vi "Data Ref FGV.vi"(5 "FIFO Idx Qs":T1, 7 "Command":T2=enum."Get", 8 "error in (no error)":errorcluster, 10 "HWOutput Length":i32, 11 "HWInput Length":i32) -> (0 "error out":errorcluster, 2 "HWOutput FIFO Index / Length":i32, 3 "HWInput FIFO Index / Length":i32)   [LabVIEW 2011, in "AIT 1553 Custom Device.lvlib"]
uses:
  AIT 1553 Custom Device.lvlib
  RT Controls/Data Ref FGV Command.ctl
  RT Controls/FIFO Idx Qs.ctl
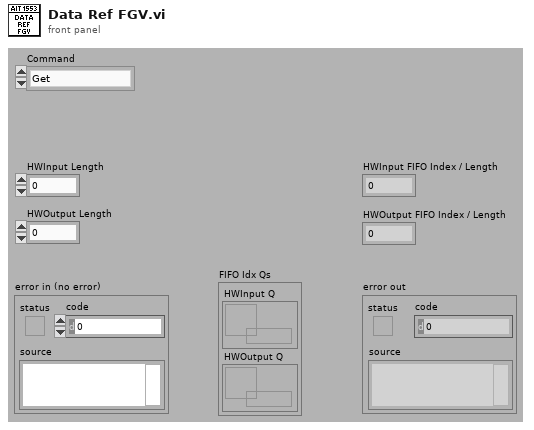
[diagram p1: front panel]
types:
  T1 = typedef "AIT 1553 Custom Device.lvlib/FIFO Idx Qs.ctl" = cluster{"HWInput Q":refnum<queue>, "HWOutput Q":refnum<queue>}
  T2 = typedef "AIT 1553 Custom Device.lvlib/Data Ref FGV Command.ctl" = enum16{"Intialize", "Get", "Update"}
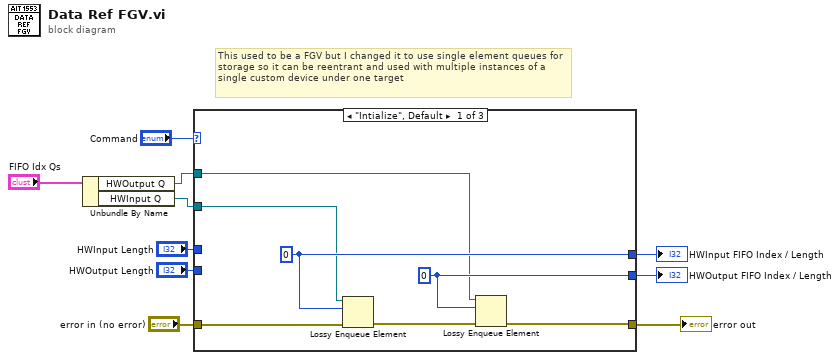
[diagram p0: block diagram]
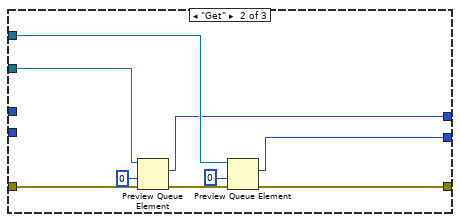
[diagram p2: hidden frame]
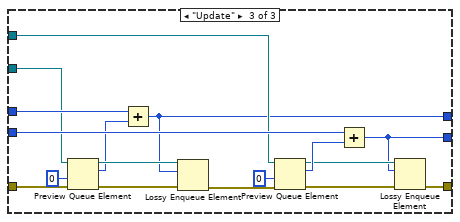
[diagram p3: hidden frame]
diagram:
  # "This used to be a FGV but I changed it to use single element queues for storage so it can be reentrant and used with multiple instances of a single custom device under one target"
  n1 = Unbundle By Name("FIFO Idx Qs") -> ("HWOutput Q"=w2:refnum<queue>, "HWInput Q"=w1:refnum<queue>)
  n2 = case shown="\"Intialize\", Default" "Command" {
    tunnel: "HWInput Length" -> [_ _ w43]
    tunnel: "HWOutput Length" -> [_ _ w42]
    tunnel: [w14 w21 w34] -> w7
    tunnel: [w13 w20 w30] -> w6
    tunnel: "error in (no error)" -> [w17 w26 w41]
    tunnel: [w16 w24 w33] -> w4
    tunnel: w1 -> [w12 w23 w39]
    tunnel: w2 -> [w11 w22 w38]
    frame "Intialize", Default {
      w13 = 0 ("index")
      w14 = 0 ("index")
      n3 = Lossy Enqueue Element(queue=w12, element=w14, error in (no error)=w17) -> (error out=w15:errorcluster)  [unwired: 3 out]
      n4 = Lossy Enqueue Element(queue=w11, element=w13, error in (no error)=w15) -> (error out=w16:errorcluster)  [unwired: 3 out]
    }
    frame "Get" {
      n5 = Preview Queue Element(queue=w23, timeout in ms (-1)=0, error in (no error)=w26) -> (element=w21:i32, error out=w25:errorcluster)  [unwired: 2 out]
      n6 = Preview Queue Element(queue=w22, timeout in ms (-1)=0, error in (no error)=w25) -> (element=w20:i32, error out=w24:errorcluster)  [unwired: 2 out]
    }
    frame "Update" {
      n7 = Preview Queue Element(queue=w39, timeout in ms (-1)=0, error in (no error)=w41) -> (queue out=w36:refnum<queue>, element=w35:i32, error out=w37:errorcluster)  [unwired: 1 out]
      n8 = Add(x=w43, y=w35) -> (x+y=w34:i32)
      n9 = Lossy Enqueue Element(queue=w36, element=w34, error in (no error)=w37) -> (error out=w29:errorcluster)  [unwired: 3 out]
      n10 = Preview Queue Element(queue=w38, timeout in ms (-1)=0, error in (no error)=w29) -> (queue out=w31:refnum<queue>, element=w32:i32, error out=w28:errorcluster)  [unwired: 1 out]
      n11 = Add(x=w42, y=w32) -> (x+y=w30:i32)
      n12 = Lossy Enqueue Element(queue=w31, element=w30, error in (no error)=w28) -> (error out=w33:errorcluster)  [unwired: 3 out]
    }
  }
  "HWInput FIFO Index / Length" <- w7
  "HWOutput FIFO Index / Length" <- w6
  "error out" <- w4
